vi "SeCrTS-DD NS Receiver Storage.vi"(11 "NOT DIS Out":T1) -> ()   [LabVIEW 2022 SP3]
uses:
  Control/SeCrTS-Notifier Ref.ctl
  Globals/SeCrTS-DD globals.vi
  <resource>/objmgr/ni.dex.rc
panel:
  out "x":u32
  out "error out":errorcluster
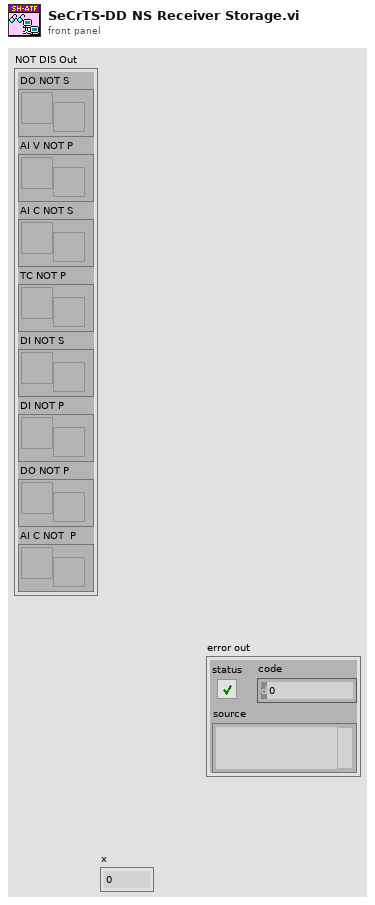
[diagram p1: front panel]
types:
  T1 = typedef "SeCrTS-Notifier Ref.ctl" = cluster{"DO NOT S":refnum<notifier>, "AI V NOT P":refnum<notifier>, "AI C NOT S":refnum<notifier>, "TC NOT P":refnum<notifier>, "DI NOT S":refnum<notifier>, "DI NOT P":refnum<notifier>, "DO NOT P":refnum<notifier>, "AI C NOT  P":refnum<notifier>}
  T2 = cluster{"In Progress":bool, "reader url":refnum<k21>, "DI P\nDI S":refnum<queue>[], "analog queue":refnum<queue>[], "NOT DIS Out":T1}
  T3 = enum16{"Initialize", "Wait for connection", "Send data", "Exit", "Receive Data"}
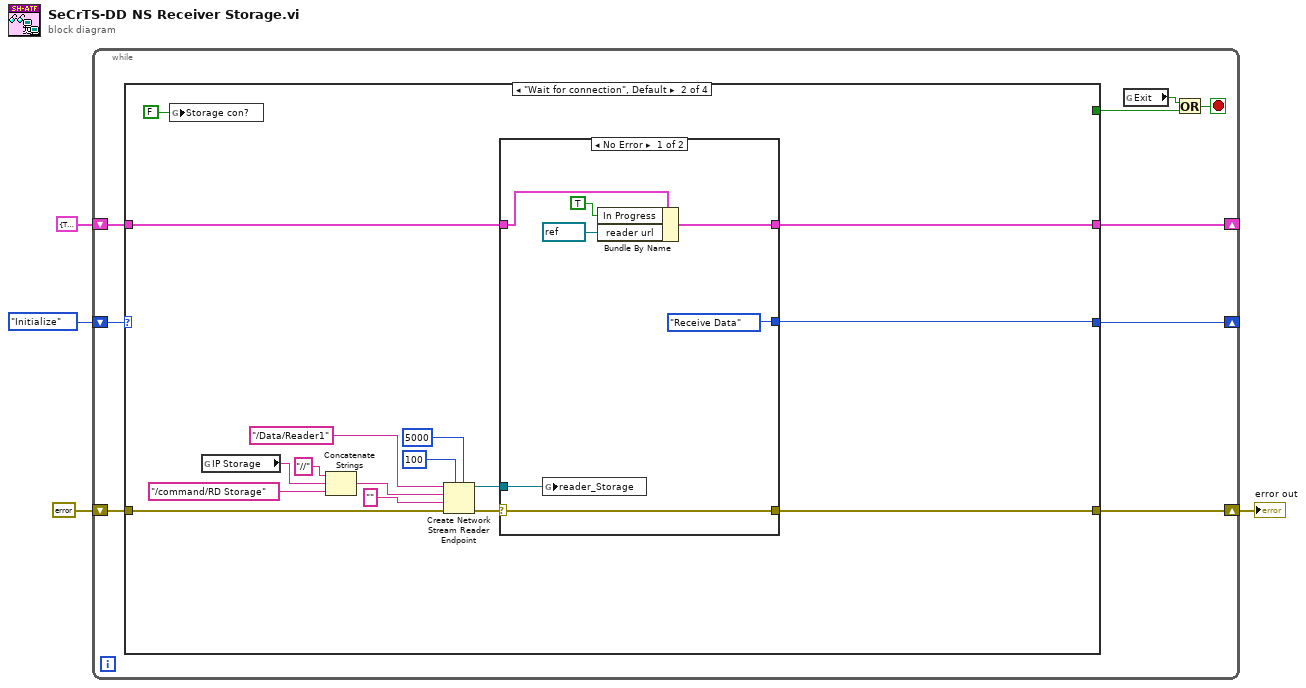
[diagram p0: block diagram]
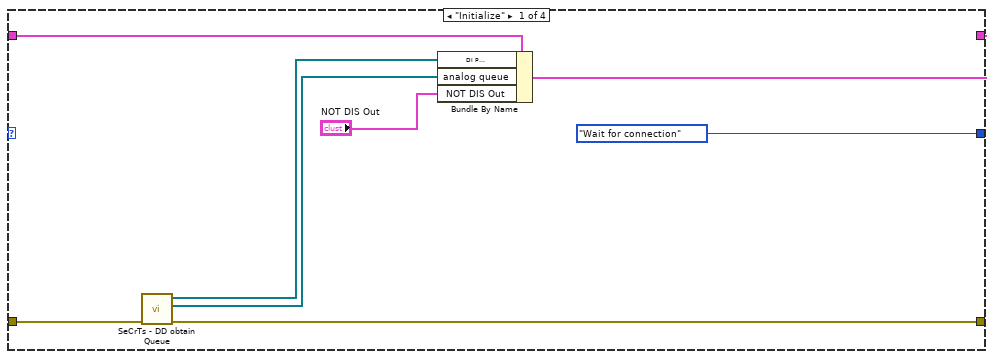
[diagram p2: hidden frame]
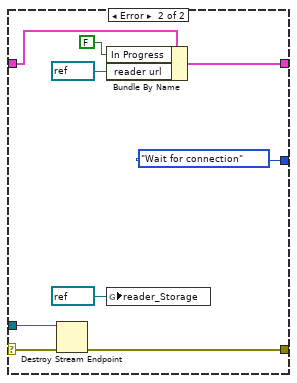
[diagram p3: hidden frame]
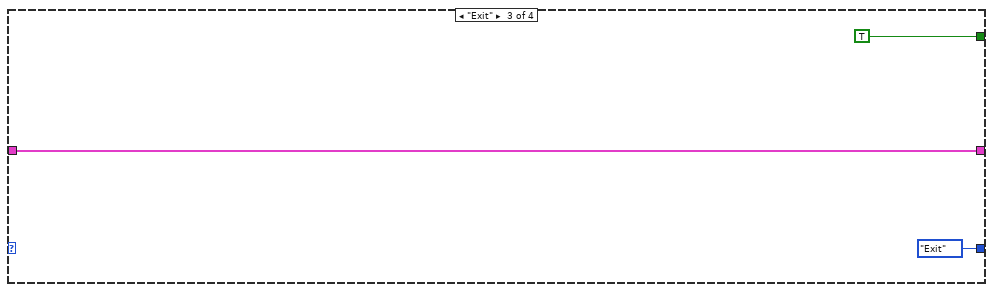
[diagram p4: hidden frame]
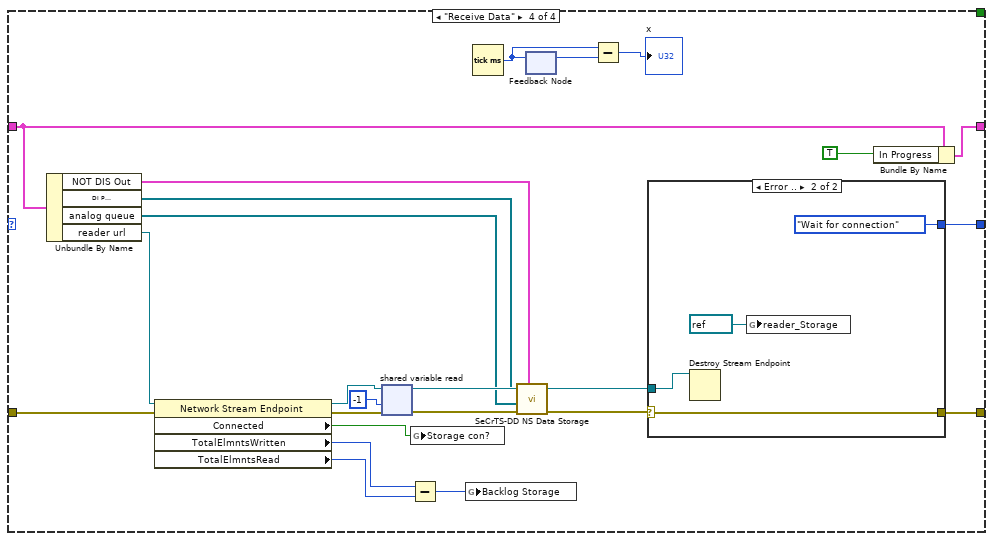
[diagram p5: hidden frame]
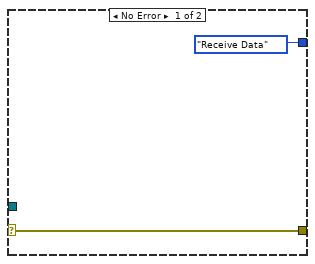
[diagram p6: hidden frame]
diagram:
  n1 = while {
    shift-right: [w11] -> _
    shift-left: T3."Initialize" -> [w13]
    shift-right: [w9] -> _
    shift-left: T2 {"In Progress"=TRUE, "reader url"="", "DI P\nDI S"=[], "analog queue"=[], "NOT DIS Out"={"DO NOT S"=refnum, "AI V NOT P"=refnum, "AI C NOT S"=refnum, "TC NOT P"=refnum, "DI NOT S"=refnum, "DI NOT P"=refnum, "DO NOT P"=refnum, "AI C NOT  P"=refnum}} -> [w10]
    shift-right: [w7] -> w2
    shift-left: errorcluster {"status"=FALSE, "code"=0, "source"=""} ("error in") -> [w8]
    stop <- w6 stop-if-true
    n2 = case shown="\"Wait for connection\", Default" w13 {
      tunnel: [_ _ TRUE _] -> w12
      tunnel: [T3."Wait for connection" w33 T3."Exit" w77] -> w11
      tunnel: w10 -> [w15 w37 w55 w66]
      tunnel: [w16 w36 w55 w78] -> w9
      tunnel: w8 -> [w20 w35 _ w79]
      tunnel: [w19 w34 _ w76] -> w7
      frame "Initialize" {
        n3 = call "SeCrTs - DD obtain Queue.vi"("error in"=w20) -> ("error out"=w19:errorcluster, "AI_V_Data P\nAI_C_Data P\nAO_Data P\nDO_Data P\nACC_Data P\nTC Data P\nDrive_A_C \nDrive_A_D\nAI_C_Data S\nDO_Data S"=w18:refnum<queue>[], "DI P\nDI S"=w17:refnum<queue>[])  [unwired: 8 in]
        n4 = Bundle By Name(cluster=w15, "DI P\nDI S"=w17, "analog queue"=w18, "NOT DIS Out"="NOT DIS Out") -> (w16:T2)
      }
      frame "Wait for connection", Default {
        n5 = global write "SeCrTS-DD globals.vi" "Storage con?"(FALSE ("Storage con?")) -> ()
        n6 = global read "SeCrTS-DD globals.vi" "IP Storage"() -> (w24:string)
        n7 = Concatenate Strings("//" ("string"), w24, "/command/RD Storage" ("reader url")) -> (w26:string)
        n8 = Create Network Stream Reader Endpoint(5:5000 ("timeout in ms (-1)"), 7:100 ("reader buffer size"), 8:w35, 9:"", 10:w26, 11:"/Data/Reader1" ("writer name")) -> (0:w30:errorcluster, 3:w31:refnum<k21>)  [unwired: 1 in]
        n9 = case shown="No Error" w30 {
          selector: w30 -> [w41 w49]
          tunnel: w37 -> [w44 w53]
          tunnel: w31 -> [w39 w50]
          tunnel: [w42 w52] -> w36
          tunnel: [w41 w48] -> w34
          tunnel: [T3."Receive Data" T3."Wait for connection"] -> w33
          frame No Error {
            n10 = global write "SeCrTS-DD globals.vi" "reader_Storage"(w39) -> ()
            n11 = Bundle By Name(cluster=w44, "In Progress"=TRUE, "reader url"=refnum<k21> refnum) -> (w42:T2)
          }
          frame Error {
            n12 = Destroy Stream Endpoint(8:w49, 11:w50) -> (0:w48:errorcluster)
            n13 = Bundle By Name(cluster=w53, "In Progress"=FALSE, "reader url"=refnum<k21> refnum) -> (w52:T2)
            n14 = global write "SeCrTS-DD globals.vi" "reader_Storage"(refnum<k21> refnum ("reader")) -> ()
          }
        }
      }
      frame "Exit" {
      }
      frame "Receive Data" {
        n15 = Unbundle By Name(w66) -> ("NOT DIS Out"=w60:T1, "DI P\nDI S"=w59:refnum<queue>[], "analog queue"=w58:refnum<queue>[], "reader url"=w57:refnum<k21>)
        n16 = property class="Network Stream Endpoint"(reference=w57, error in=w79) -> (reference out=w74:refnum<k21>, error out=w73:errorcluster, "Connected"=w72:bool, "TotalElmntsWritten"=w64:u64, "TotalElmntsRead"=w63:u64)
        n17 = shared-variable-read(w74, w73, -1 ("timeout ms (-1)")) -> (w65:refnum<k21>, w62:errorcluster)  [unwired: 2 out]
        n18 = Subtract(x=w64, y=w63) -> (x-y=w67:u64)
        n19 = global write "SeCrTS-DD globals.vi" "Storage con?"(w72) -> ()
        n20 = global write "SeCrTS-DD globals.vi" "Backlog Storage"(w67) -> ()
        n21 = Tick Count (ms)() -> (millisecond timer value=w70:u32)
        n22 = call "SeCrTS-DD NS Data Storage.vi"("NOT DIS Out"=w60, "error in"=w62, "AI_V_Data P\nAI_C_Data P\nAO_Data P\nDO_Data P\nACC_Data P\nTC Data P\nDrive_A_C \nDrive_A_D\nAI_C_Data S\nDO_Data S"=w58, "DI P\nDI S"=w59) -> ("error out"=w61:errorcluster)  [unwired: 7 in]
        n23 = feedback #1() -> (w71:u32)  [unwired: 1 in]
        n24 = feedback-in #1(w70) -> ()
        n25 = Subtract(x=w70, y=w71) -> (x-y=→"x":u32)
        n26 = case shown="Error .." w61 {
          selector: w61 -> [w81 w82]
          tunnel: [w81 w82] -> w76
          tunnel: [T3."Receive Data" T3."Wait for connection"] -> w77
          tunnel: w65 -> [_ w84]
          frame No Error {
          }
          frame Error {
            n27 = Destroy Stream Endpoint(11:w84) -> ()  [unwired: 1 in, 1 out]
            n28 = global write "SeCrTS-DD globals.vi" "reader_Storage"(refnum<k21> refnum ("reader_Storage")) -> ()
          }
        }
        n29 = Bundle By Name(cluster=w66, "In Progress"=TRUE) -> (w78:T2)
      }
    }
    n30 = global read "SeCrTS-DD globals.vi" "Exit"() -> (w5:bool)
    n31 = Or(x=w5, y=w12) -> (x .or. y?=w6:bool)
  }
  "error out" <- w2
